vi "user32_IsWindowVisible.vi"(0 "hWnd":u32, 11 "错误输入（无错误）":errorcluster) -> (4 "dup hWnd":u32, 6 "IsWindowVisible?":bool, 15 "错误输出":errorcluster)   [LabVIEW 2011]
doc: "该函数获得给定窗口的可视状态。"
uses:
  user32.dll
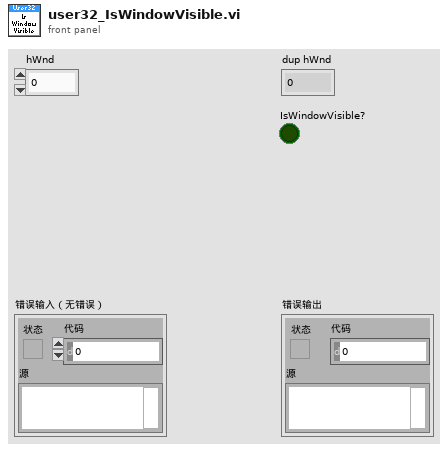
[diagram p1: front panel]
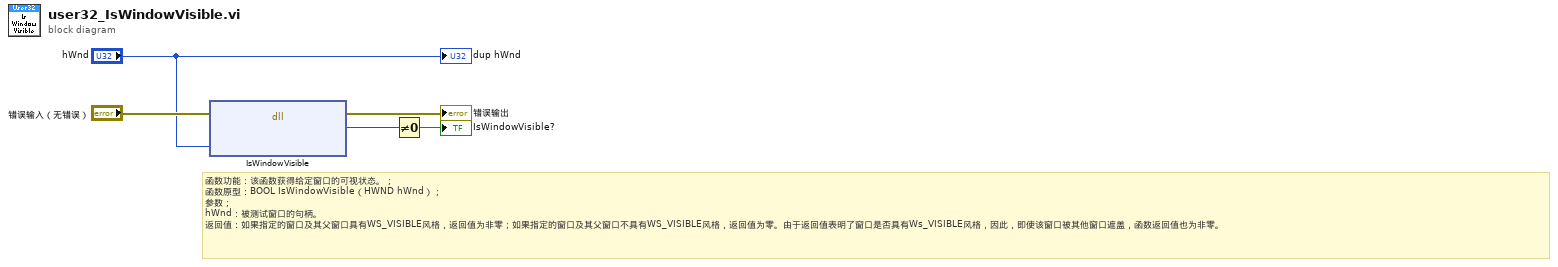
[diagram p0: block diagram]
diagram:
  # "函数功能：该函数获得给定窗口的可视状态。；\n函数原型：BOOL IsWindowVisible（HWND hWnd）；\n参数；\nhWnd：被测试窗口的句柄。\n返回值：如果指定的窗口及其父窗口具有WS_VISIBLE风格，返回值为非零；如果指定的窗口及其父窗口不具有WS_VISIBLE风格，返回值为零。由于返回值表明了窗口是否具有Ws_VISIBLE风格，因此，即使该窗口被其他窗口遮盖，函数返回值也为非零。"
  n1 = dll-call lib="user32.dll" fn="IsWindowVisible"(error in="错误输入（无错误）", "hWnd"="hWnd") -> (error out=→"错误输出":errorcluster, "Bool"=w2:u8)  [unwired: 3 in, 1 out]
  n2 = Not Equal To 0?(x=w2) -> (x != 0?=→"IsWindowVisible?":bool)
  "dup hWnd" <- "hWnd"
